vi "waitOnIRQ.vi"(8 "error in (no error)":errorcluster, 10 "Timeout":i32, 11 "OuterLoopClockIRQ in":refnum<class "OuterLoopClockIRQ.lvclass">) -> (0 "error out":errorcluster, 1 "TimedOut":bool, 2 "IRQs":i32[](array[numeric]), 3 "OuterLoopClockIRQ out":refnum<class "OuterLoopClockIRQ.lvclass">)   [LabVIEW 2016, in "OuterLoopClockIRQ.lvclass"]
uses:
  OuterLoopClockIRQ.lvclass
  OuterLoopClockIRQ.lvclass/OuterLoopClockIRQ.ctl
  FPGA/FPGA.lvclass
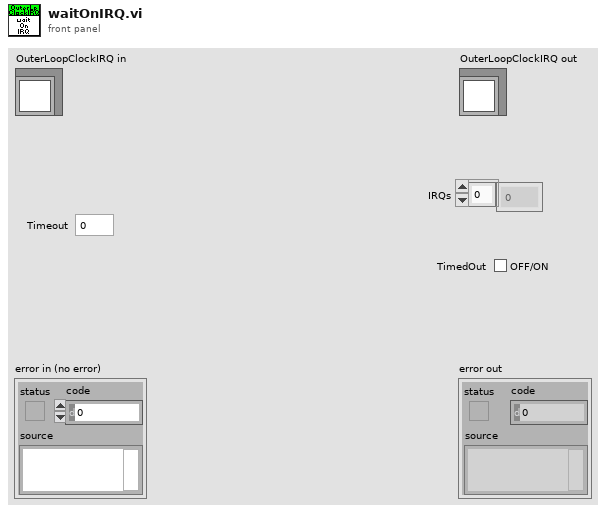
[diagram p1: front panel]
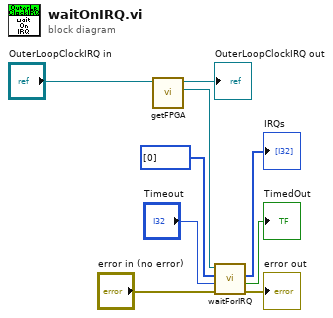
[diagram p0: block diagram]
diagram:
  n1 = call "getFPGA.vi"("OuterLoopClockIRQ in"="OuterLoopClockIRQ in") -> ("FPGA"=w8:refnum<class "FPGA.lvclass">, "OuterLoopClockIRQ out"=→"OuterLoopClockIRQ out":refnum<class "OuterLoopClockIRQ.lvclass">)  [unwired: 9 in]
  n2 = call "waitForIRQ.vi"("error in (no error)"="error in (no error)", "Timeout (ms)"="Timeout", "IRQs in"=i32[] [0], "FPGA in"=w8) -> ("error out"=→"error out":errorcluster, "TimedOut"=→"TimedOut":bool, "IRQs out"=→"IRQs":i32[])  [unwired: 4 in, 1 out]
